vi "UniPend.vi"(0 "initial alpha":dbl=3.1416, 1 "initial velocity alpha":dbl, 7 "Torque (Tau)":dbl, 12 "friction coefficient 1":dbl=0.02, 14 "Amplifier Gain":dbl(slide)=0.4 scale=0.0..3.0) -> (6 "alpha1":dbl=0.11676928692181643)   [LabVIEW 2012]
uses:
  <vilib>/Simulation/Implementation/XNodeFramework/SimXNode/SimX.xnode
  <vilib>/Simulation/ContinuousLinear/Implementation/NILVSim Integrator new.llb/SIM Integrator (scalar).vi
  <vilib>/ptbypt/Time Domain.llb/Unwrap Phase PtByPt.vi
  <vilib>/ptbypt/NI_PtbyPt.lvlib
panel:
  in  "Gravitational Force (m/s^2)":dbl=9.81
  in  "Moment of Inetia of the frame wrt to center of mass (Ifg)":dbl=20.0
  in  "Distance from center of wheel to center of mass (Rf)":dbl=0.463
  in  "Radius of Wheel (Rw)":dbl=0.2032
  in  "Moment of Inertia wrt center of mass (Iwg)":dbl=0.0812
  in  "Mass of Frame (mf)":dbl=25.0
  in  "Mass of Bottom Wheel (mw)":dbl=7.645
  # "Legend: \nC.G.  - Center of Gravity\nl       - Length (m)\nJ      - Moment of Inertia (kg(m^2)\nM     - Mass (kg)"
  # "Derived Parameters"
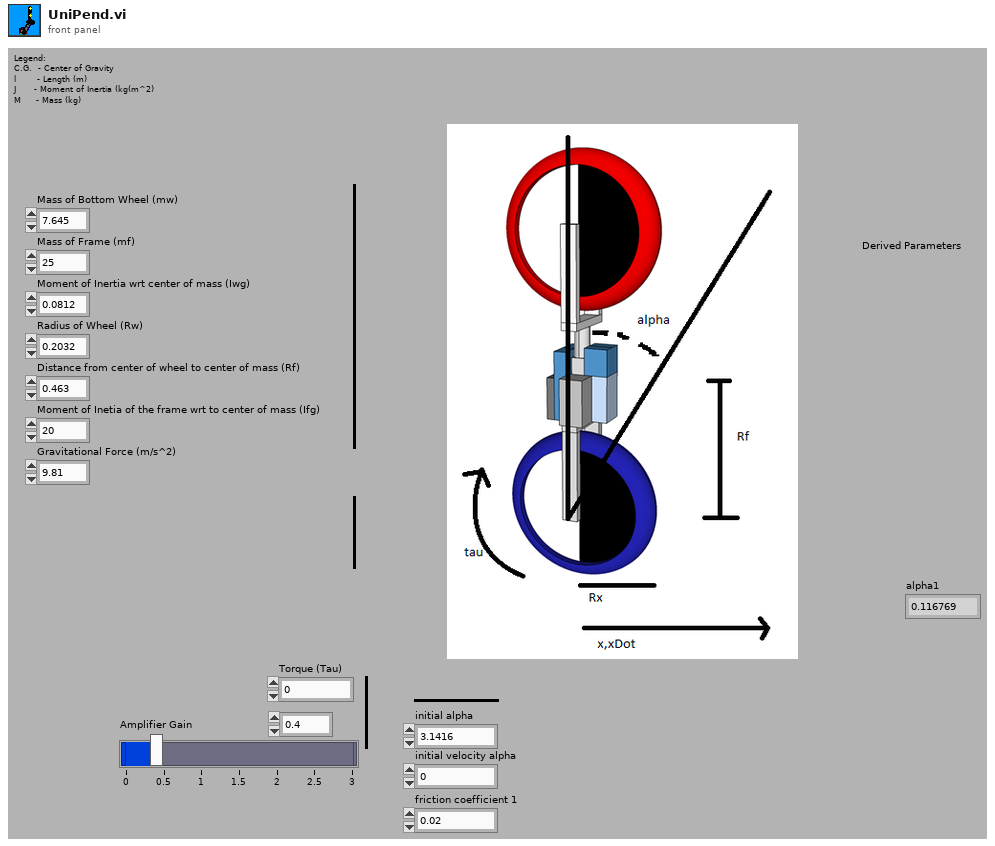
[diagram p1: front panel]
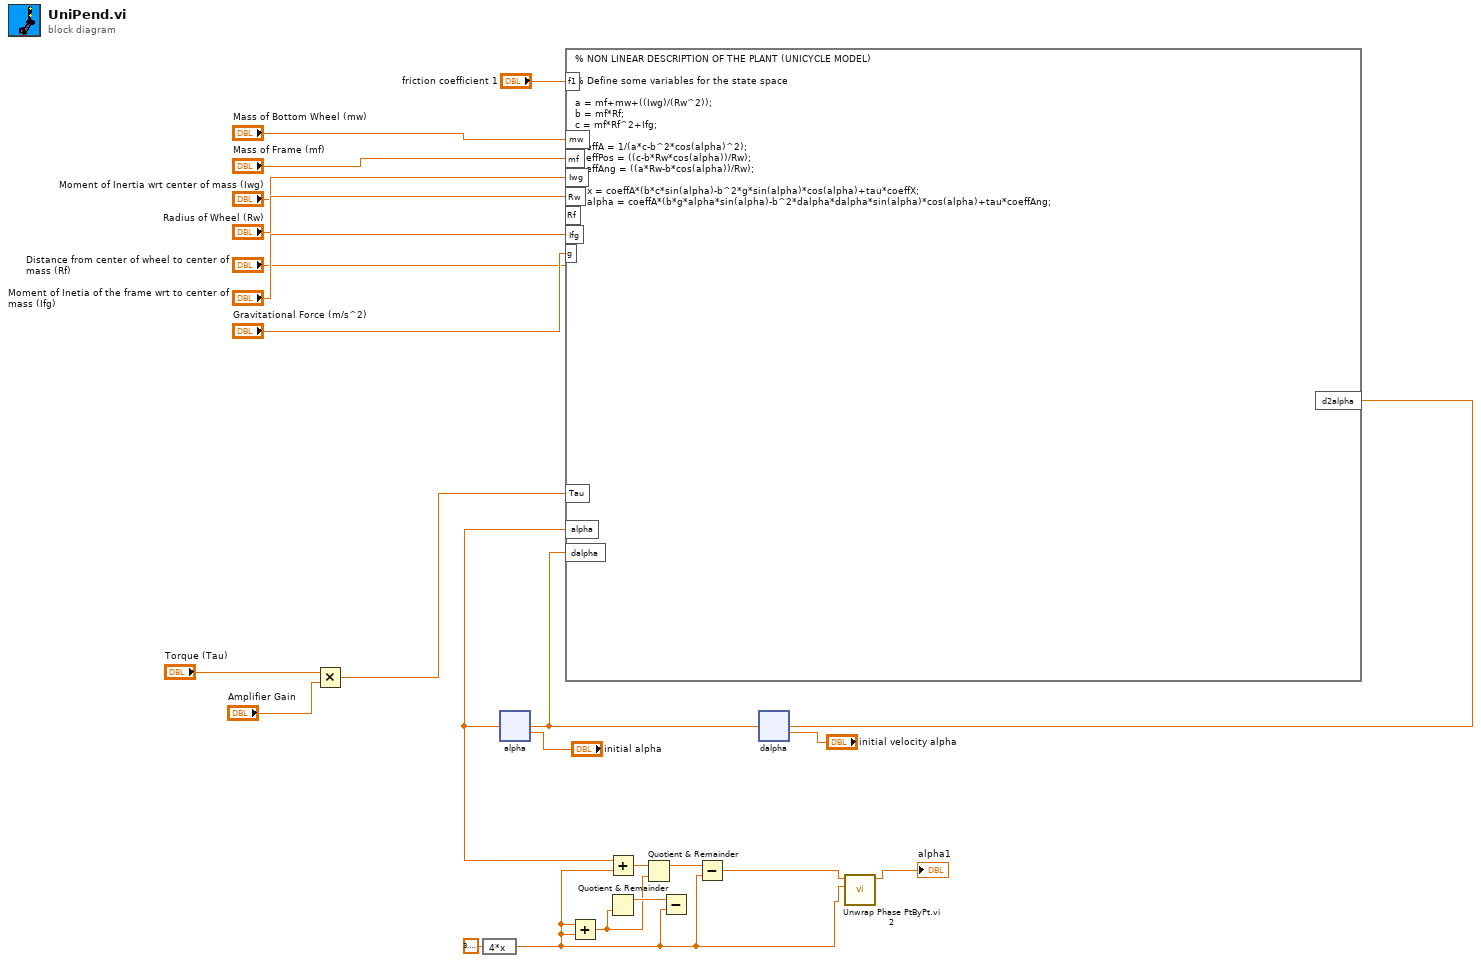
[diagram p0: block diagram]
diagram:
  n1 = Multiply ("Multiply 8")(x="Torque (Tau)", y="Amplifier Gain") -> (x*y=w22:dbl)
  n2 = expression code="4*x"(3.141592653589793 ("Constant")) -> (w8:dbl)
  n3 = Add ("Add 6")(x=w8, y=w8) -> (x+y=w11:dbl)
  n4 = Quotient & Remainder(y=w11) -> (x-y*floor(x/y)=w16:dbl)  [unwired: 1 in, 1 out]
  n5 = Subtract(x=w16, y=w8) -> ()  [unwired: 1 out]
  n6 = xnode "alpha"("input"=w17, "initial condition"="initial alpha") -> ("output"=w13:dbl)  [unwired: 8 in, 2 out]
  n7 = Add ("Add 5")(x=w13, y=w8) -> (x+y=w14:dbl)
  n8 = Quotient & Remainder ("Quotient & Remainder 2")(x=w14, y=w11) -> (x-y*floor(x/y)=w15:dbl)  [unwired: 1 out]
  n9 = Subtract ("Subtract 2")(x=w15, y=w8) -> (x-y=w10:dbl)
  n10 = call "Unwrap Phase PtByPt.vi 2"("wrap base"=w8, "phase"=w10) -> ("unwrapped phase"=→"alpha1":dbl)  [unwired: 9 in]
  n11 = formula code="% NON LINEAR DESCRIPTION OF THE PLANT (UNICYCLE MODEL)\n\n% Define some variables for the state space\n\na = mf+mw+((Iwg)/(Rw^2));\nb = mf*Rf;\nc = mf*Rf^2+Ifg;\n\ncoeffA = 1/(a*c-b^2*cos(alpha)^2);\ncoeffPos = ((c-b*Rw*cos(alpha))/Rw);\ncoeffAng = ((a*Rw-b*cos(alpha))/Rw);\n\nd2x = coeffA*(b*c*sin(alpha)-b^2*g*sin(alpha)*cos(alpha)+tau*coeffX;\nd2alpha = coeffA*(b*g*alpha*sin(alpha)-b^2*dalpha*dalpha*sin(alpha)*cos(alpha)+tau*coeffAng;"("Tau"=w22, "alpha"=w13, "dalpha"=w17, "f1"="friction coefficient 1", "mw"="Mass of Bottom Wheel (mw)", "mf"="Mass of Frame (mf)", "Iwg"="Moment of Inertia wrt center of mass (Iwg)", "Rw"="Radius of Wheel (Rw)", "Rf"="Distance from center of wheel to center of mass (Rf)", "Ifg"="Moment of Inetia of the frame wrt to center of mass (Ifg)", "g"="Gravitational Force (m/s^2)") -> ("d2alpha"=w24:dbl)
  n12 = xnode "dalpha"("input"=w24, "initial condition"="initial velocity alpha") -> ("output"=w17:dbl)  [unwired: 8 in, 2 out]
